vi "Initialize.vi"(8 "error in (no error)":errorcluster, 11 "Device in":refnum<class "RS232_Device.lvclass">) -> (0 "error out":errorcluster, 3 "Device out":refnum<class "RS232_Device.lvclass">)   [LabVIEW 2023, in "RS232_Device.lvclass"]
uses:
  RS232_Device.lvclass
  D:/SamparkProdLine/subVIs/DAQ Device/Modbus_Device/DAQ_Device.lvclass
  RS232_Device.lvclass/RS232_Device.ctl
  <vilib>/Instr/_visa.llb/VISA Configure Serial Port (Instr).vi
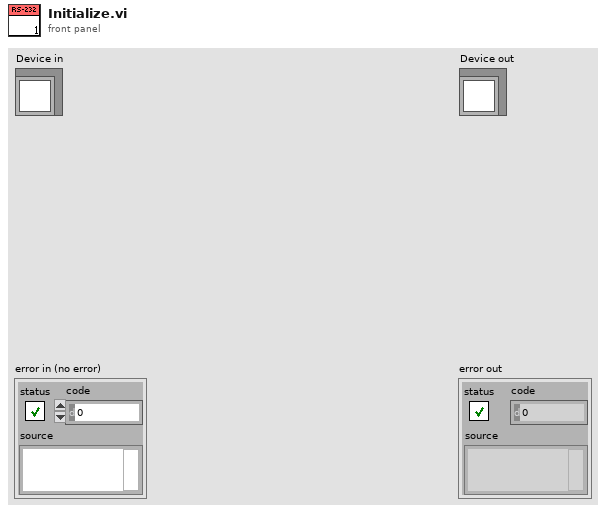
[diagram p1: front panel]
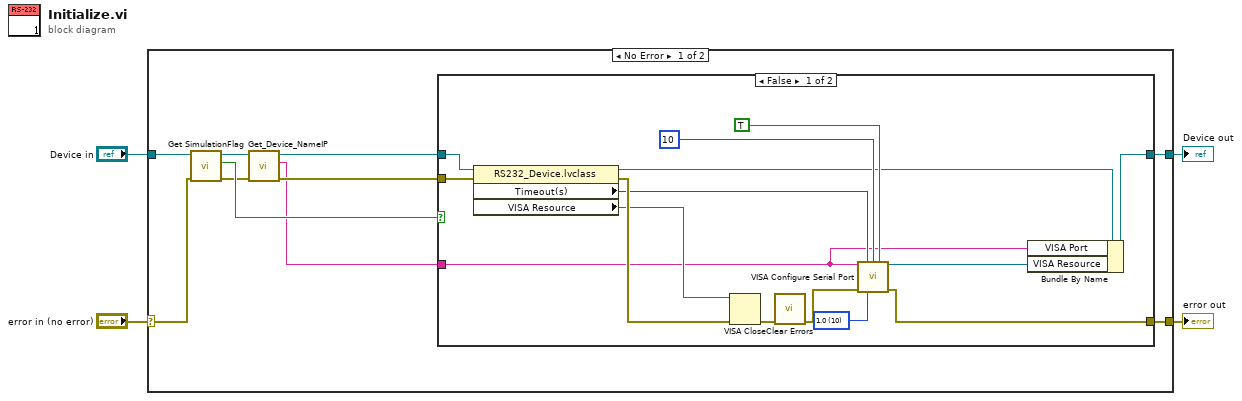
[diagram p0: block diagram]
diagram:
  n1 = case shown="No Error" "error in (no error)" {
    selector: "error in (no error)" -> [w10 w33]
    tunnel: [w13 w33] -> w3
    tunnel: [w14 w32] -> w1
    tunnel: "Device in" -> [w12 w32]
    frame No Error {
      n2 = call-dynamic "Get SimulationFlag.vi"("error in (no error)"=w10, "Device in"=w12) -> ("error out"=w6:errorcluster, "Simulation?"=w11:bool, "Device out"=w9:refnum<class "RS232_Device.lvclass">)  [unwired: 7 in]
      n3 = call-dynamic "Get_Device_NameIP.vi"("error in (no error)"=w6, "Device in"=w9) -> ("error out"=w7:errorcluster, "Device Address"=w5:string, "Device out"=w8:refnum<class "RS232_Device.lvclass">)  [unwired: 4 in, 3 out]
      n4 = case shown="False" w11 {
        tunnel: w8 -> [w19 w31]
        tunnel: [w28 w31] -> w14
        tunnel: [w21 w30] -> w13
        tunnel: w7 -> [w16 w30]
        tunnel: w5 -> [w15 _]
        frame False {
          w26 = u16 10 items=["1.0"=10, "1.5"=15, "2.0"=20] ("stop bits (10: 1 bit)")
          n5 = property class="RS232_Device.lvclass"(reference=w19, error in=w16) -> (reference out=w20:refnum<class "RS232_Device.lvclass">, error out=w29:errorcluster, "Timeout(s)"=w18:i32, "VISA Resource"=w17:refnum<visa-resource-name>)
          n6 = VISA Close(VISA resource name=w17, error in (no error)=w29) -> (error out=w27:errorcluster)
          n7 = call <vilib>:"Clear Errors.vi"("error in (no error)"=w27) -> ("error out"=w25:errorcluster)  [unwired: 5 in, 1 out]
          n8 = call-poly "VISA Configure Serial Port"("VISA resource name"=w15, "timeout (10sec)"=w18, "termination char\n(0xA = '\\n' = LF)"=u8 10 ("termination char\n(0xA = '\\n' = LF)"), "Enable Termination\nChar (T)"=TRUE ("Enable Termination\nChar (T)"), "error in (no error)"=w25, "stop bits (10: 1 bit)"=w26) -> ("VISA resource name out"=w24:refnum<visa-resource-name>, "error out"=w21:errorcluster)  [unwired: 8 in]
          n9 = Bundle By Name(cluster=w20, "VISA Port"=w15, "VISA Resource"=w24) -> (w28:refnum<class "RS232_Device.lvclass">)
        }
        frame True {
        }
      }
    }
    frame Error {
    }
  }
  "error out" <- w3
  "Device out" <- w1
